vi "Obtain UserPrefs.vi"(8 "error in (no error)":errorcluster) -> (0 "error out":errorcluster, 3 "PrefsDB out":refnum<class "PrefsDB.lvclass">)   [LabVIEW 2020, in "User Prefs.lvlib" / "PrefsDB.lvclass"]
uses:
  PrefsDB.lvclass
  PrefsDB.lvclass/PrefsDB.ctl
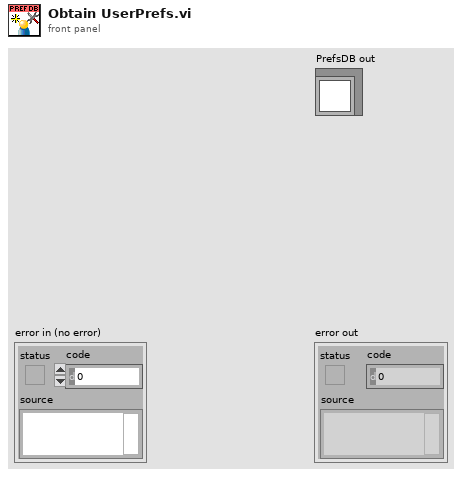
[diagram p1: front panel]
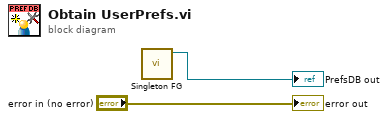
[diagram p0: block diagram]
diagram:
  n1 = call "Singleton FG.vi"() -> ("PrefsDB"=→"PrefsDB out":refnum<class "PrefsDB.lvclass">)  [unwired: 11 in]
  "error out" <- "error in (no error)"
